vi "rvc Rotate Matrix X-axis.vi"(6 "angle unit":u16(ring)=1 items=["degree", "radians"], 10 "angle":dbl, 11 "rotation matrix in":T1) -> (3 "rotation matrix":T1)   [LabVIEW 2013]
uses:
  <vilib>/Analysis/Matrix/Datatypes/RealMatrix.ctl
  <vilib>/Analysis/Matrix/NI_Matrix.lvlib
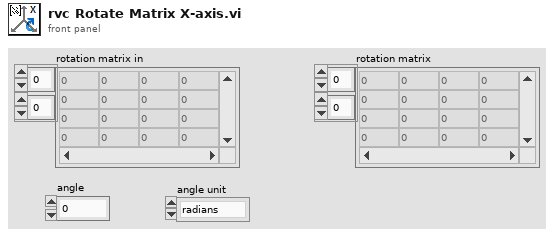
[diagram p1: front panel]
types:
  T1 = typedef "NI_Matrix.lvlib/RealMatrix.ctl" = dbl[][]
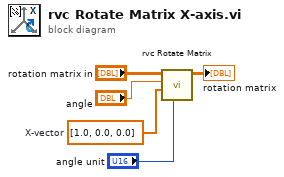
[diagram p0: block diagram]
diagram:
  w3 = dbl[] [1.0, 0.0, 0.0]  # X-vector
  n1 = call "rvc Rotate Matrix.vi"("angle unit"="angle unit", "vector"=w3, "angle"="angle", "rotation matrix in"="rotation matrix in") -> ("rotation matrix"=→"rotation matrix":T1)  [unwired: 7 in]
